vi "Child Address.vi"(6 "Unified Actor Alias":string, 7 "Actor in":refnum<class "Actor.lvclass">) -> (0 "Error out":errorcluster, 2 "Address":refnum<event-registration>)   [LabVIEW 2020, in "jettl.lvlib" / "Read Unified Actor.lvlib"]
uses:
  Read Unified Actor.lvlib
  Msg/Msg.lvclass
  Actor/Actor.lvclass
  Msg Contents/Msg Contents.lvclass
  jettl.lvlib
  Unified Actor Relation.ctl
  Teller.ctl
  Msg.ctl
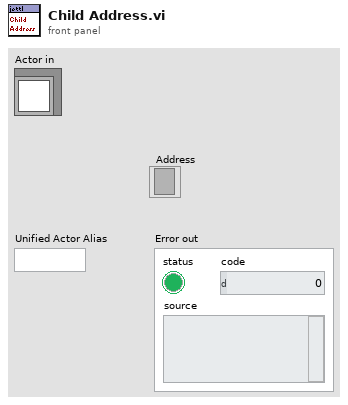
[diagram p1: front panel]
types:
  T1 = typedef "jettl.lvlib/Unified Actor.ctl" = cluster{"Msgs":T2, "Leaf":bool, "Edge Actors":refnum<class "Actor.lvclass">[], "Mid Actors":refnum<class "Actor.lvclass">[], "Core Actors":refnum<class "Actor.lvclass">[], "Root":bool, "Alias":string, "Transport":refnum<user-event>, "Address":refnum<event-registration>, "This VI":refnum<vi>}
  T2 = typedef "jettl.lvlib/Msgs.ctl" = cluster{"Inbound":T3, "Outbound":T3, "Implemented":T3, "Tell Init":T3, "Tell Init Self":T3, "Tell Init Parent":T3, "Tell Init Child":T3, "Tell Forward":T3, "Tell Forward Self":T3, "Tell Forward Parent":T3, "Tell Forward Child":T3}
  T3 = typedef "jettl.lvlib/Msg Set.ctl" = set{refnum<class "Msg.lvclass">}
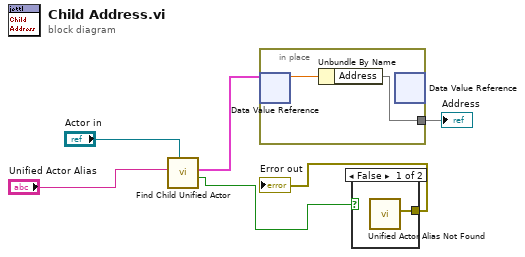
[diagram p0: block diagram]
diagram:
  n1 = call "Find Child Unified Actor.vi"("Actor in"="Actor in", "Unified Actor Alias"="Unified Actor Alias") -> ("Found"=w2:bool, "Child Unified Actor"=w4:T1)  [unwired: 8 in]
  n2 = in-place {
    in-place-border: [w7] -> w3
    n3 = in-place-dvr #1(w4) -> (w8:dbl)  [unwired: 1 out]
    n4 = Unbundle By Name(w8) -> ("Address"=w7)
    n5 = in-place-dvr #1() -> ()  [unwired: 1 in, 2 out]
  }
  "Address" <- w3
  n6 = case shown="False" w2 {
    tunnel: [w9 _] -> w1
    frame False {
      n7 = call "Unified Actor Alias Not Found.vi"() -> ("Error"=w9:errorcluster)  [unwired: 11 in]
    }
    frame True {
    }
  }
  "Error out" <- w1
